vi "ReceiveRigidBodies.vi"() -> ()   [LabVIEW 2011]
uses:
  <vilib>/FPGAPlugInAG/sbRIO-9636/niLvFpga_Open_sbRIO-9636.vi
  <vilib>/rvi/interface/common/dynamic/niFpgaDynamicAddResources.vi
  <vilib>/FPGAPlugInAG/Dynamic/niLvFpga_Run_Dynamic.vi
  <vilib>/Utility/error.llb/Error Cluster From Error Code.vi
  <vilib>/rvi/errors/niLvFpgaAdjustHostInterfaceError.vi
  <vilib>/FPGAPlugInAG/Dynamic/niLvFpga_Close_Dynamic.vi
  <vilib>/rvi/interface/nirviOpenFPGA/nirviOpenFPGA.xnode
  FPGA Bitfiles/TreadmillControl_FPGATarget_Exercise2_CF30559D.lvbitx
  FPGA/FPGA.vi
  <vilib>/rvi/interface/nirviMethod/nirviMethod.xnode
  <vilib>/rvi/interface/nirviReadWriteControl/nirviReadWriteControl.xnode
  <vilib>/rvi/interface/nirviCloseFPGA/nirviCloseFPGA.xnode
  <vilib>/FPGAPlugInAG/Dynamic/niLvFpga_ReadFifo_Dynamic.vi
  <vilib>/rvi/errors/niLvFpgaMergeErrorWithErrorCode.vi
  NiFpgaLv.dll
  <vilib>/rvi/interface/Simulation/niFpgaSimulationCallBeginRW.vi
  <vilib>/FPGAPlugInAG/Dynamic/niLvFpga_WriteFifo_Dynamic.vi
panel:
  out "Packet":u8[](array[numeric])
  in  "RobotEnable":bool
  in  "UseTreadmillSpeed":bool
  in  "SpeedCommand":fxp<+/-,20,5>
  out "FilteredRPM":fxp<+/-,33,18>=-0.09429931640625
  in  "PIDSetpoint":fxp<+/-,16,18>=200.0
  in  "UsePID":bool
  in  "DriveEnable":bool
  out "Vl":dbl=34.80019912307633
  out "Vr":dbl=-7.165531849511732
  in  "Ks":dbl=0.5
  in  "d":dbl=0.7
  in  "Kt":dbl=5.0
  in  "Ky":dbl=5.0
  in  "Vt":dbl
  in  "Kx":dbl=2.0
  in  "SetOffset":bool
  out "State":dbl[](array[numeric])=[-6.90760612487793, 5.977581024169922, 0.017523400485515594]
  out "ToggleTime":u32=9
  in  "Decimation":i32=1
  out "ReadData":u8[](array[numeric])=[56] format="%x"
  in  "stop":bool
  out "error out":errorcluster={"status"=TRUE, "code"=56, "source"="UDP Read in ReceiveRigidBodies.vi"}
  in  "port":u16=1511
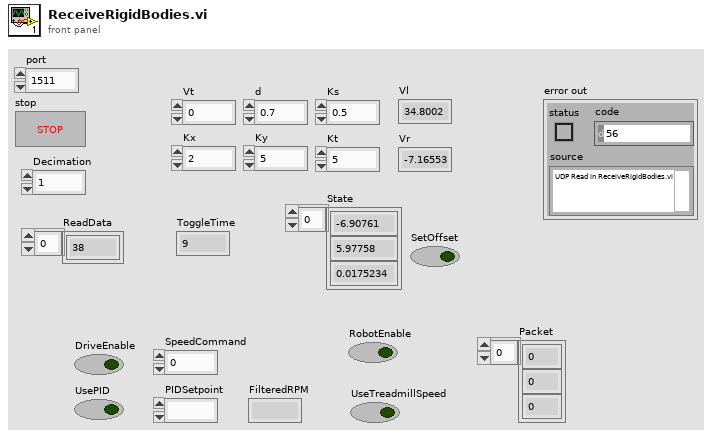
[diagram p1: front panel]
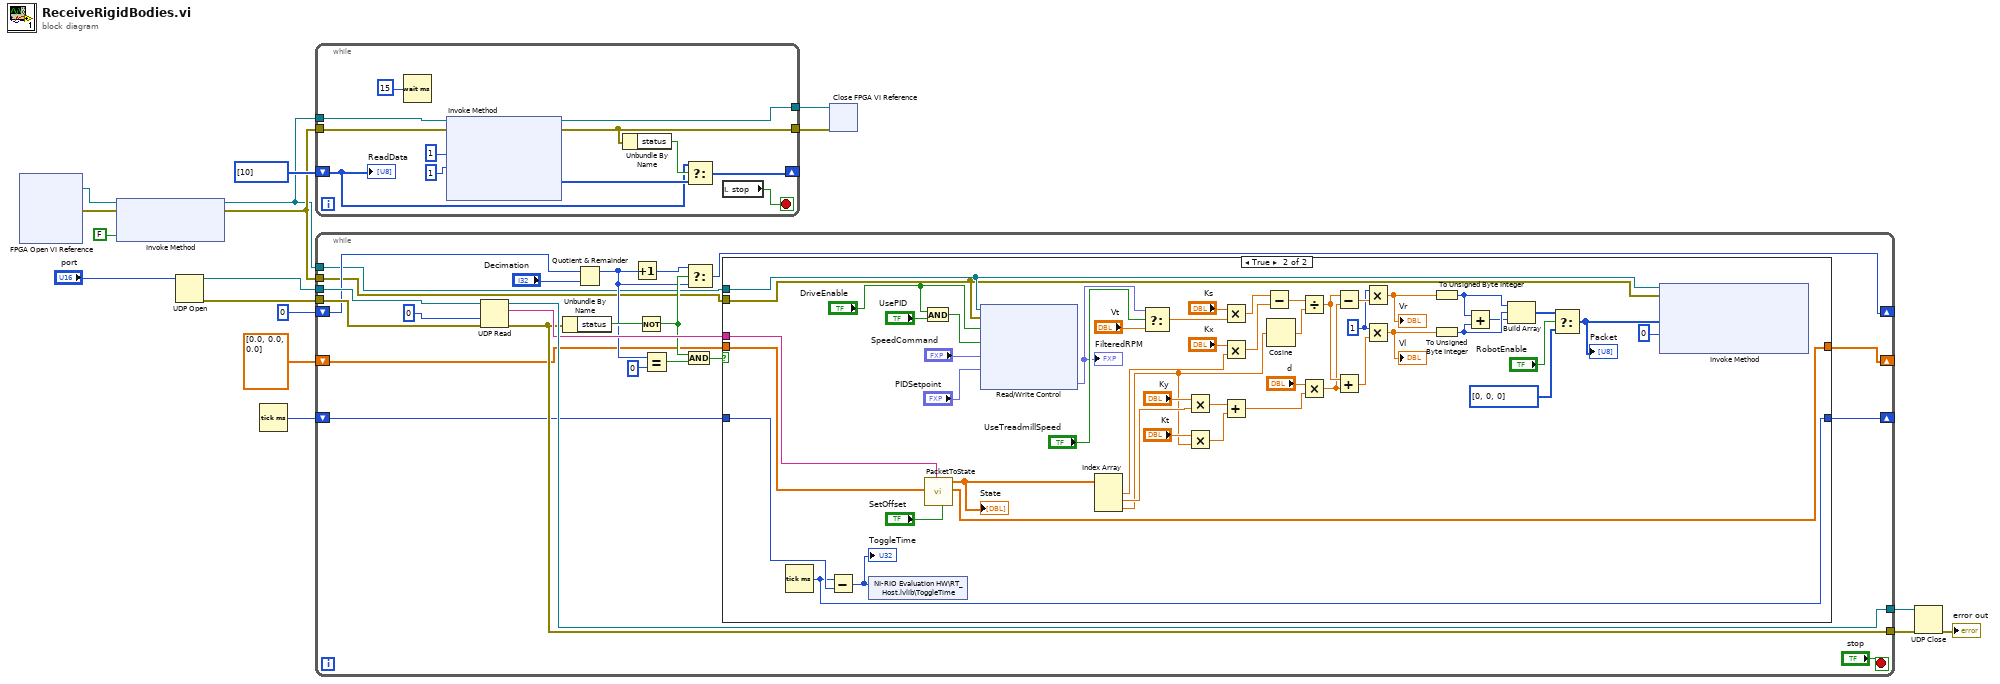
[diagram p0: block diagram]
diagram:
  n1 = xnode "FPGA Open VI Reference"() -> ("FPGA VI Reference Out"=w11:refnum<k20>, "error out"=w10:errorcluster)  [unwired: 2 in]
  n2 = xnode "Invoke Method"("FPGA VI Reference In"=w11, "error in"=w10, "Wait Until Done (F)"=FALSE) -> ("FPGA VI Reference Out"=w2:refnum<k20>, "error out"=w3:errorcluster)
  n3 = UDP Open(11:"port") -> (port=w14:refnum<k16>, 0:w13:errorcluster)  [unwired: 4 in, 1 out]
  n4 = Tick Count (ms)() -> (millisecond timer value=w4:u32)
  n5 = while {
    tunnel: w2 -> [w28]
    tunnel: w3 -> [w29]
    tunnel: [w25] -> w8
    tunnel: [w24] -> w7
    shift-right: [w21] -> _
    shift-left: u8[] [10] ("WriteData") -> [w19]
    stop <- w23 stop-if-true
    n6 = Wait (ms)(milliseconds to wait=u32 15) -> ()  [unwired: 1 out]
    n7 = xnode "Invoke Method"("FPGA VI Reference In"=w28, "error in"=w29, "Number of Elements"=u32 1 ("ReadElements"), "Timeout (ms)"=1 ("ReadTimeout")) -> ("FPGA VI Reference Out"=w25:refnum<k20>, "error out"=w24:errorcluster, "Data"=w20:u8[])  [unwired: 1 out]
    n8 = Unbundle By Name(w24) -> ("status"=w22:bool)
    n9 = Select(t=w19, s=w22, f=w20) -> (s? t:f=w21:u8[])
    n10 = local read "stop"() -> (w23:bool)
    "ReadData" <- w19
  }
  n11 = while {
    tunnel: [w51] -> w17
    tunnel: [w46] -> w16
    tunnel: w14 -> [w49]
    tunnel: w13 -> [w48]
    shift-right: [w37] -> _
    shift-left: 0 ("y") -> [w43]
    shift-right: [w35] -> _
    shift-left: w4 -> [w36]
    tunnel: w3 -> [w34]
    tunnel: w2 -> [w33]
    shift-right: [w31] -> _
    shift-left: dbl[] [0.0, 0.0, 0.0] -> [w30]
    stop <- "stop" stop-if-true
    n12 = UDP Read(connection ID=w49, timeout ms (25000)=0, 8:w48) -> (data out=w47:string, error out=w46:errorcluster, 3:w51:refnum<k16>)  [unwired: 1 in, 2 out]
    n13 = Unbundle By Name(w46) -> ("status"=w45:bool)
    n14 = Quotient & Remainder(x=w43, y="Decimation") -> (x-y*floor(x/y)=w39:i32)  [unwired: 1 out]
    n15 = Increment(x=w39) -> (x+1=w38:i32)
    n16 = Not(x=w45) -> (.not. x?=w40:bool)
    n17 = Equal?(x=w39, y=0) -> (x = y?=w41:bool)
    n18 = And(x=w40, y=w41) -> (x .and. y?=w32:bool)
    n19 = Select(t=w38, s=w40, f=w39) -> (s? t:f=w37:i32)
    n20 = case shown="True" w32 {
      tunnel: w47 -> [_ w103]
      tunnel: w36 -> [w54 w100]
      tunnel: [w54 w99] -> w35
      tunnel: w34 -> [_ w76]
      tunnel: w33 -> [_ w77]
      tunnel: [w53 w97] -> w31
      tunnel: w30 -> [w53 w98]
      frame False {
      }
      frame True {
        w55 = 1
        n21 = Tick Count (ms)() -> (millisecond timer value=w99:u32)
        n22 = Subtract(x=w99, y=w100) -> (x-y=w101:u32)
        "ToggleTime" <- w101
        n23 = shared-variable "NI-RIO Evaluation HW\\RT_Host.lvlib\\ToggleTime"(w101) -> ()  [unwired: 1 in, 1 out]
        n24 = And(x="DriveEnable", y="UsePID") -> (x .and. y?=w71:bool)
        n25 = call "PacketToState.vi"("SetOffset"="SetOffset", "DataPacket"=w103, "OffsetsIn"=w98) -> ("OffsetsOut"=w97:dbl[], "State"=w95:dbl[])  [unwired: 7 in]
        "State" <- w95
        n26 = xnode "Read/Write Control"("FPGA VI Reference In"=w77, "error in"=w76, "DriveEnable"="DriveEnable", "UsePID"=w71, "SpeedCommand"="SpeedCommand", "PIDSetpoint"="PIDSetpoint") -> ("FilteredRPM"=w68:fxp<+/-,33,18>)  [unwired: 2 out]
        "FilteredRPM" <- w68
        n27 = Index Array(array=w95) -> (element #1=w86:dbl, element #2=w94:dbl, element #3=w89:dbl)  [unwired: 3 in]
        n28 = Select(t=w68, s="UseTreadmillSpeed", f="Vt") -> (s? t:f=w58:dbl)
        n29 = Multiply(x="Ky", y=w94) -> (x*y=w85:dbl)
        n30 = Multiply(x="Kt", y=w89) -> (x*y=w84:dbl)
        n31 = Multiply(x="Ks", y=w58) -> (x*y=w56:dbl)
        n32 = Multiply(x="Kx", y=w86) -> (x*y=w91:dbl)
        n33 = Add(x=w85, y=w84) -> (x+y=w82:dbl)
        n34 = Subtract(x=w56, y=w91) -> (x-y=w90:dbl)
        n35 = Cosine(x=w89) -> (cos(x)=w88:dbl)
        n36 = Divide(x=w90, y=w88) -> (x/y=w83:dbl)
        n37 = Multiply(x="d", y=w82) -> (x*y=w80:dbl)
        n38 = Subtract(x=w83, y=w80) -> (x-y=w79:dbl)
        n39 = Add(x=w83, y=w80) -> (x+y=w78:dbl)
        n40 = Multiply(x=w55, y=w79) -> (x*y=w67:dbl)
        "Vr" <- w67
        n41 = Multiply(x=w55, y=w78) -> (x*y=w66:dbl)
        "Vl" <- w66
        n42 = To Unsigned Byte Integer(number=w67) -> (unsigned 8bit integer=w65:u8)
        n43 = To Unsigned Byte Integer(number=w66) -> (unsigned 8bit integer=w64:u8)
        n44 = Add(x=w65, y=w64) -> (x+y=w63:u8)
        n45 = Build Array(w65, w64, w63) -> (w62:u8[])
        n46 = Select(t=w62, s="RobotEnable", f=u8[] [0, 0, 0]) -> (s? t:f=w60:u8[])
        "Packet" <- w60
        n47 = xnode "Invoke Method"("FPGA VI Reference In"=w77, "error in"=w76, "Data"=w60, "Timeout (ms)"=0 ("WriteTimeout")) -> ()  [unwired: 3 out]
      }
    }
  }
  n48 = xnode "Close FPGA VI Reference"("FPGA VI Reference In"=w8, "error in"=w7) -> ()  [unwired: 1 out]
  n49 = UDP Close(connection ID=w17, 8:w16) -> (error out=→"error out":errorcluster)  [unwired: 1 out]
